vi "Save INI.vi"(8 "error in (no error)":errorcluster, 11 "HAL Editor in":refnum<class "HAL Editor.lvclass">) -> (0 "error out":errorcluster, 3 "HAL Editor out":refnum<class "HAL Editor.lvclass">)   [LabVIEW 2012, in "HAL Config.lvlib" / "HAL Editor.lvclass"]
uses:
  HAL Editor.lvclass
  build/ppl/lv-hal.lvlibp/HAL Manager/HAL Manager.lvclass
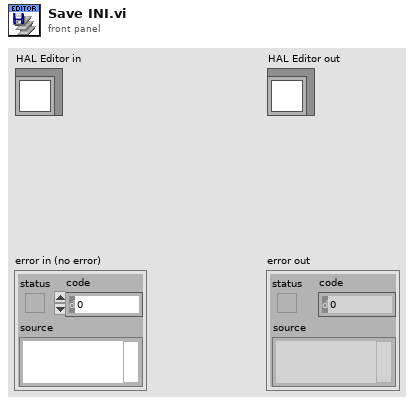
[diagram p1: front panel]
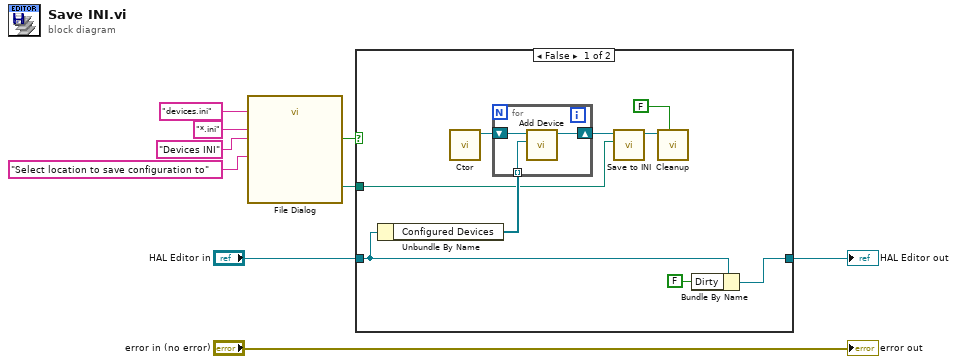
[diagram p0: block diagram]
diagram:
  n1 = call "File Dialog"("prompt"="Select location to save configuration to" ("pattern label"), "default name"="devices.ini", "pattern (all files)"="*.ini", "pattern label"="Devices INI") -> ("selected path"=w1:path, "cancelled"=w4:bool)  [unwired: 8 in, 2 out]
  n2 = case shown="False" w4 {
    tunnel: "HAL Editor in" -> [w18 w22]
    tunnel: [w17 w22] -> w2
    tunnel: w1 -> [w12 _]
    frame False {
      n3 = Unbundle By Name(w18) -> ("Configured Devices"=w14:refnum<class "Device.lvclass">[])
      n4 = call "Ctor.vi"() -> ("HAL Manager out"=w15:refnum<class "HAL Manager.lvclass">)  [unwired: 10 in, 1 out]
      n5 = for {
        shift-right: [w20] -> w13
        shift-left: w15 -> [w21]
        tunnel: w14 -> [w19] mode=indexing
        n6 = call "Add Device.vi"("Device Model"=w19, "HAL Manager in"=w21) -> ("HAL Manager out"=w20:refnum<class "HAL Manager.lvclass">)  [unwired: 7 in, 2 out]
      }
      n7 = call "Save to INI.vi"("INI Path"=w12, "HAL Manager in"=w13) -> ("HAL Manager out"=w11:refnum<class "HAL Manager.lvclass">)  [unwired: 8 in, 1 out]
      n8 = call "Cleanup.vi"("Cleanup Devices? (T)"=FALSE, "HAL Manager in"=w11) -> ()  [unwired: 9 in, 1 out]
      n9 = Bundle By Name(cluster=w18, "Dirty"=FALSE) -> (w17:refnum<class "HAL Editor.lvclass">)
    }
    frame True {
    }
  }
  "HAL Editor out" <- w2
  "error out" <- "error in (no error)"
